vi "Auto Tune.vi"() -> ()   [LabVIEW 2022 SP3]
uses:
  Control_AutoTune.ctl
  <vilib>/Analysis/baseanly.llb/Mean (DBL).vi
  <vilib>/Analysis/NI_AALBase.lvlib
panel:
  in  "Cancel Current Aquisition":bool
  out "XY Graph":cluster{"X":dbl, "Y":dbl}[](graph)=[{"X"=0.0, "Y"=0.49504944043821886}]
  out "Enum":T1
  in  "Channels to read":tag="Dev1/ai2,Dev1/ai3"
  in  "Time per aquisition (s)":dbl
  in  "Sampling Rate":dbl
  out "Best Value":dbl
  out "Max":dbl=0.49504944043821886
  in  "Increment Amount":dbl=5.0
  in  "Lower Value":dbl
  in  "Upper Value":dbl=1000.0
  in  "Start Auto Tune":bool
  in  "stop":bool
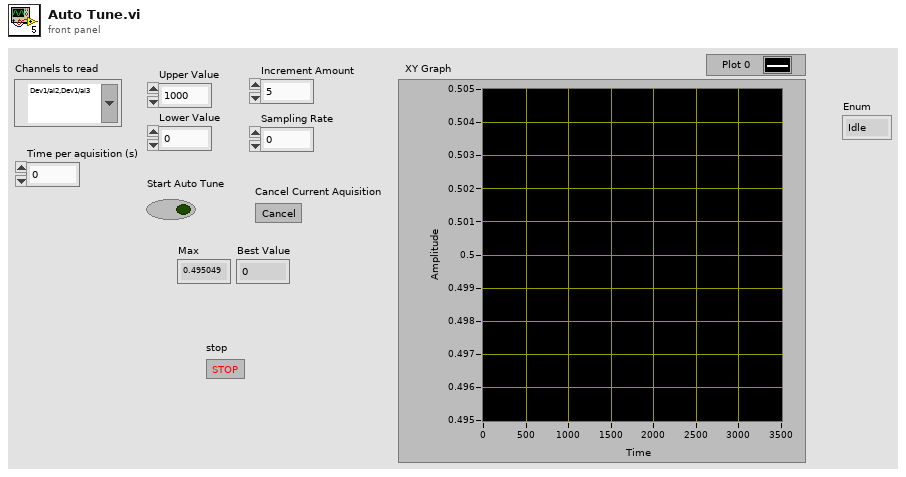
[diagram p1: front panel]
types:
  T1 = typedef "Control_AutoTune.ctl" = enum16{"Idle", "Read DAQ and Store ", "Move to Next Point", "Auto Tune"}
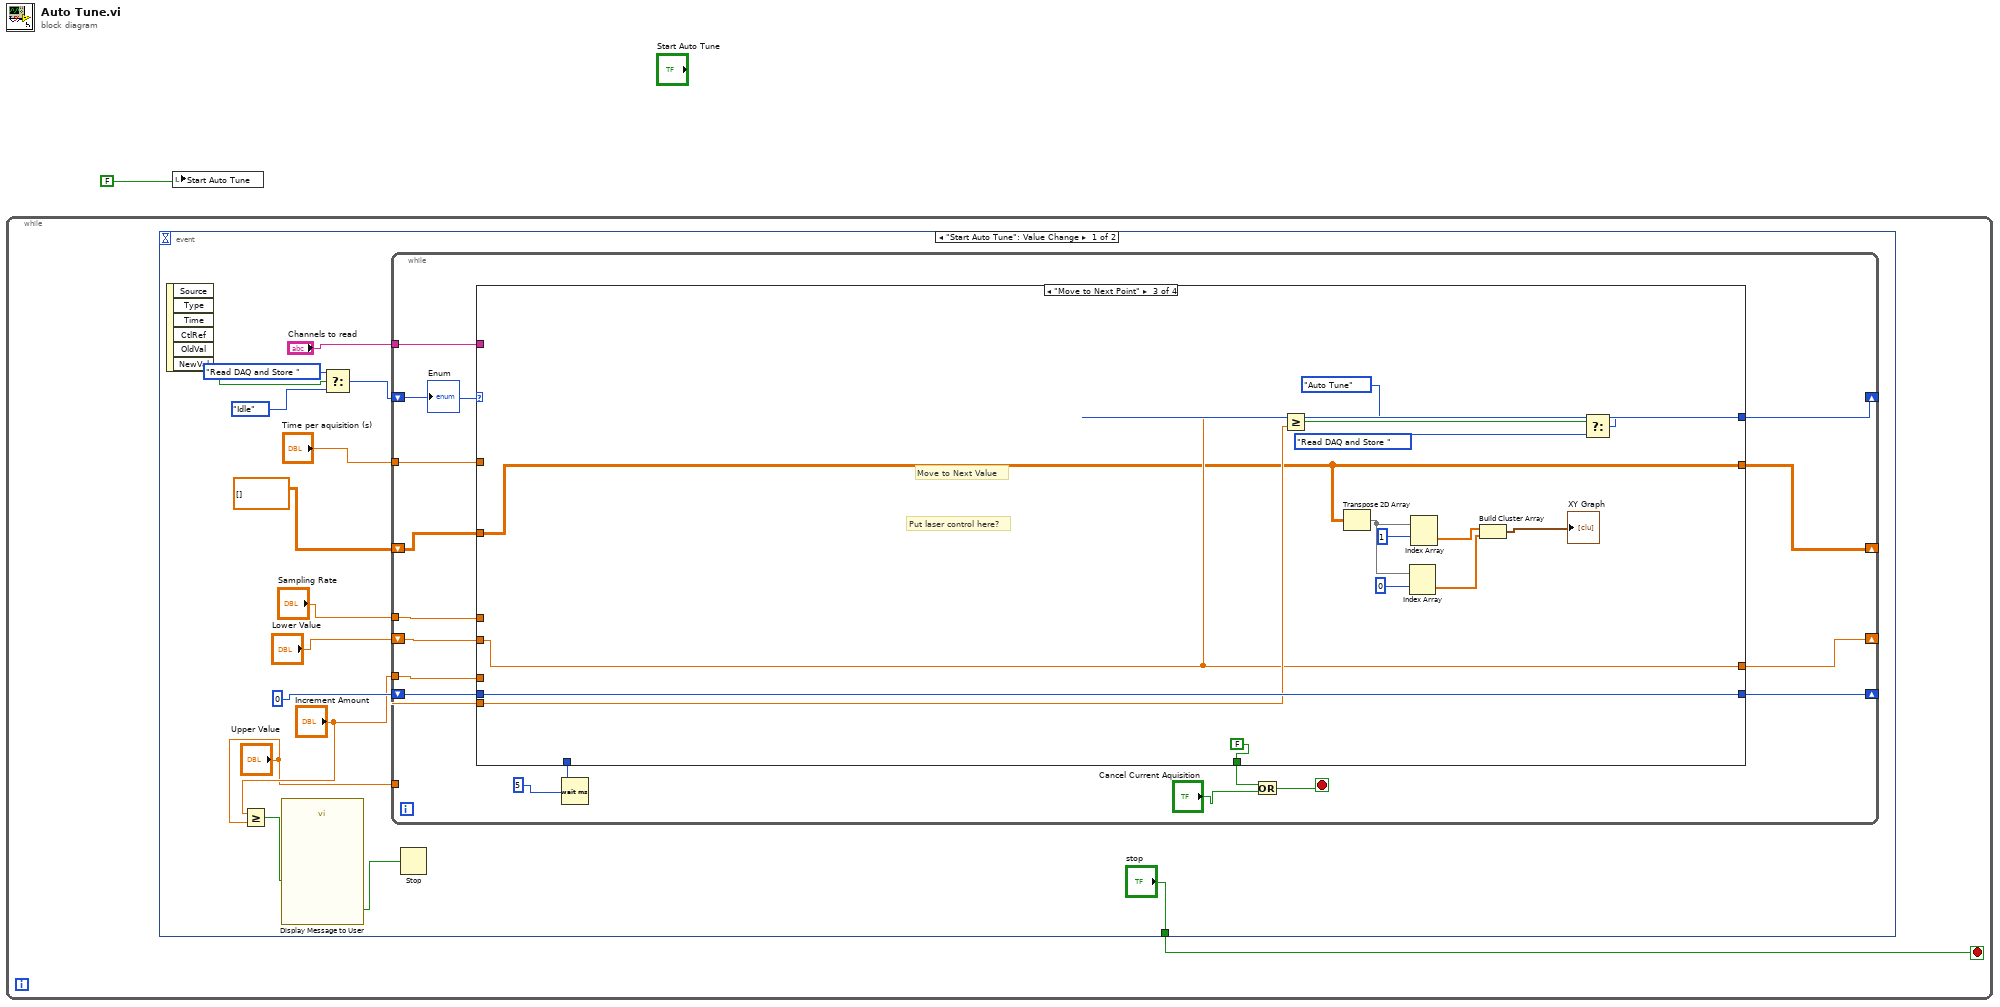
[diagram p0: block diagram]
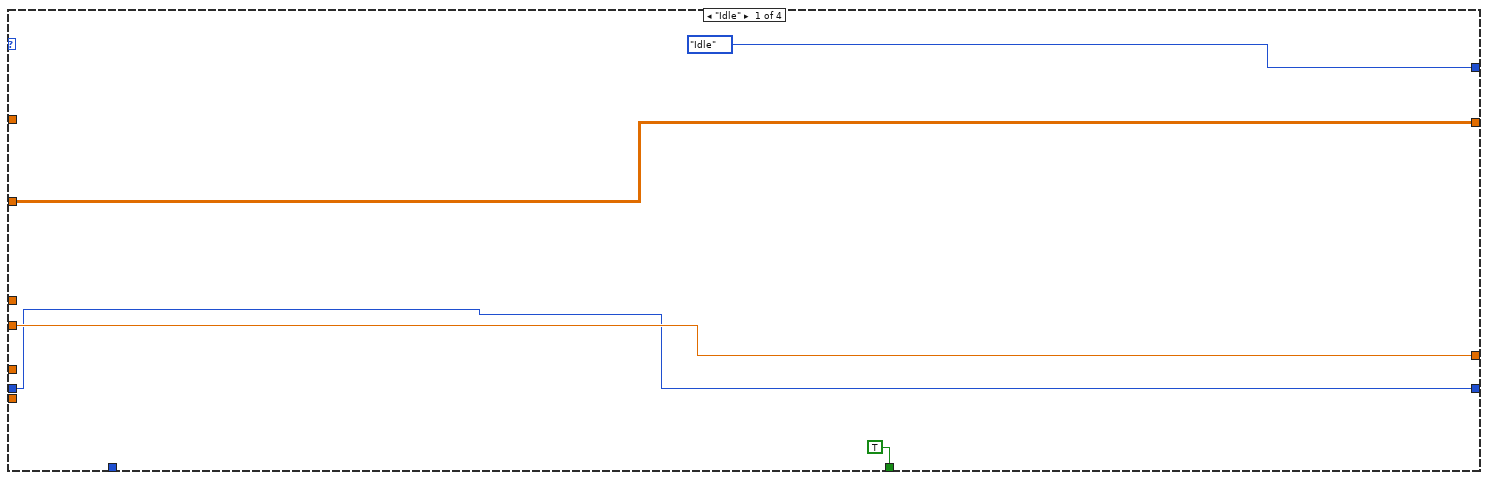
[diagram p2: hidden frame]
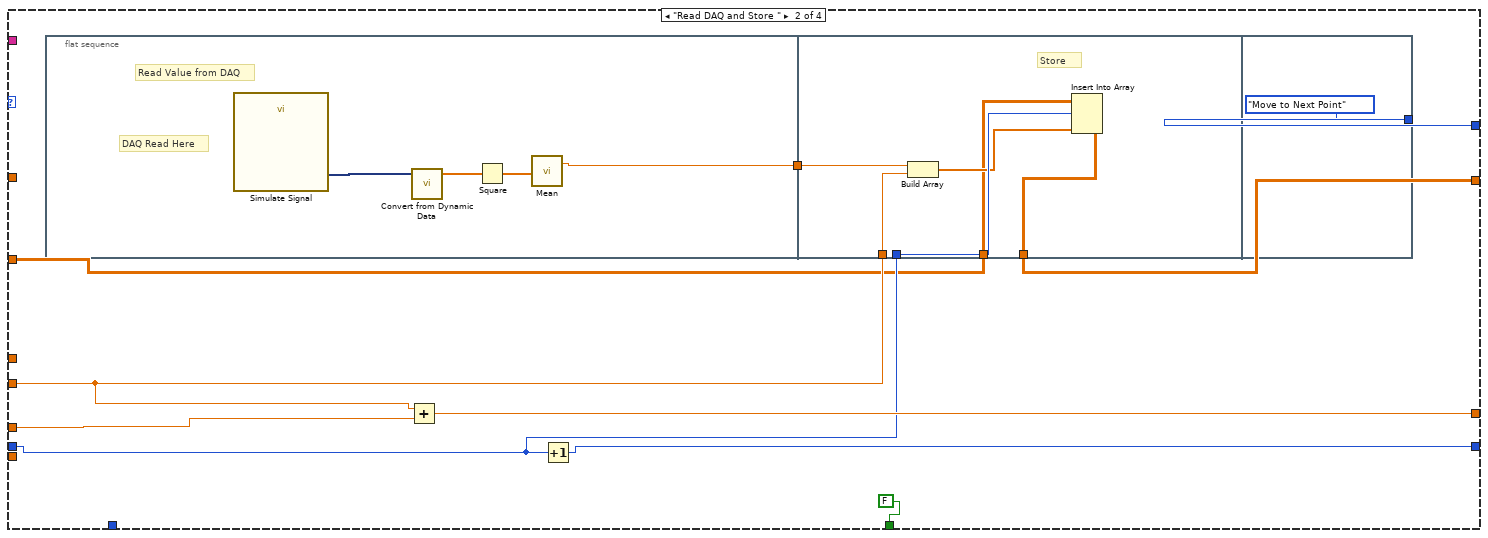
[diagram p3: hidden frame]
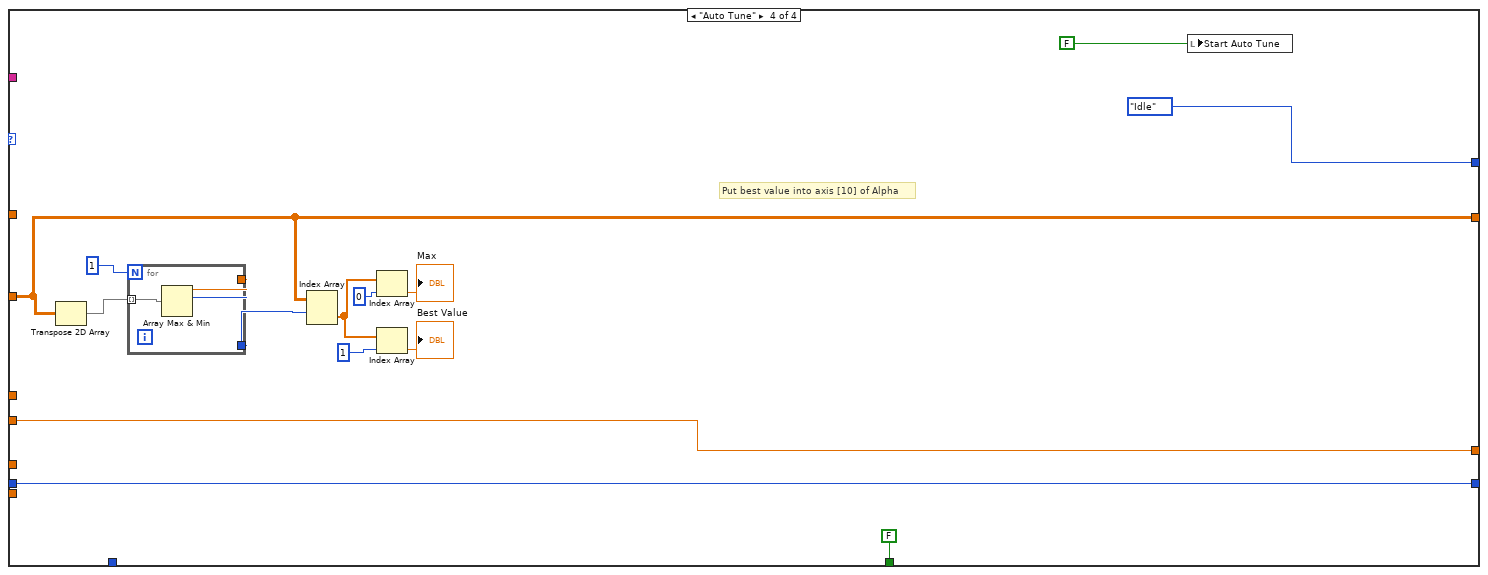
[diagram p4: hidden frame]
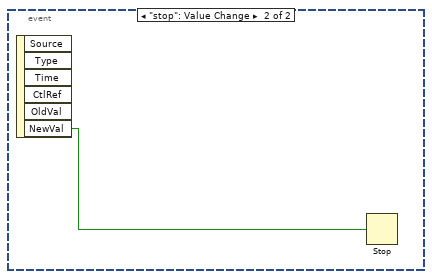
[diagram p5: hidden frame]
diagram:
  n1 = while {
    stop <- w2 stop-if-true
    n2 = event shown="[0] \"Start Auto Tune\": Value Change" {
      selector: _ -> [_ _]
      dyn-events: _ -> [_ _]
      timeout: _ -> [_ _]
      tunnel: ["stop" _] -> w2
      event "Start Auto Tune": Value Change {
        n3 = event-data() -> ("NewVal"=w7:bool)  [unwired: 1 in, 5 out]
        n4 = Greater Or Equal?(x="Increment Amount", y="Upper Value") -> (x >= y?=w6:bool)
        n5 = call "Display Message to User"("Enable"=w6) -> ("OK"=w11:bool)  [unwired: 9 in, 1 out]
        n6 = Select(t=Control_AutoTune."Read DAQ and Store ", s=w7, f=Control_AutoTune."Idle") -> (s? t:f=w8:T1)
        n7 = while {
          shift-right: [w34] -> _
          shift-left: w8 -> [w25]
          shift-right: [w32] -> _
          shift-left: dbl[][] [] -> [w31]
          tunnel: "Increment Amount" -> [w30]
          tunnel: "Upper Value" -> [w21]
          tunnel: "Time per aquisition (s)" -> [w28]
          tunnel: "Sampling Rate" -> [w27]
          tunnel: "Channels to read" -> [w26]
          shift-right: [w24] -> _
          shift-left: 0 -> [w23]
          shift-right: [w22] -> _
          shift-left: "Lower Value" -> [w29]
          stop <- w19 stop-if-true
          w33 = 5
          n8 = case shown="\"Move to Next Point\"" w25 {
            tunnel: [Control_AutoTune."Idle" w46 w72 Control_AutoTune."Idle"] -> w34
            tunnel: w33 -> [_ _ _ _]
            tunnel: [w39 w40 w65 w84] -> w32
            tunnel: w31 -> [w39 w41 w65 w84]
            tunnel: w30 -> [_ w49 _ _]
            tunnel: w29 -> [w38 w47 w69 w77]
            tunnel: w28 -> [_ _ _ _]
            tunnel: w27 -> [_ _ _ _]
            tunnel: w26 -> [_ _ _ _]
            tunnel: [w35 w44 w75 w78] -> w24
            tunnel: w23 -> [w35 w42 w75 w78]
            tunnel: [w38 w45 w69 w77] -> w22
            tunnel: w21 -> [_ _ w70 _]
            tunnel: [TRUE FALSE FALSE FALSE] -> w20
            frame "Idle" {
            }
            frame "Read DAQ and Store " {
              n9 = flat-sequence {
                tunnel: [w53] -> w48
                tunnel: w48 -> [w59]
                tunnel: w47 -> [w58]
                tunnel: w42 -> [w57]
                tunnel: w41 -> [w55]
                tunnel: [w54] -> w40
                tunnel: [Control_AutoTune."Move to Next Point"] -> w46
                frame #0 {
                  # "DAQ Read Here"
                  # "Read Value from DAQ"
                  n10 = call "Simulate Signal"() -> ("Sine"=w52:dynamicdata)  [unwired: 14 in, 1 out]
                  n11 = call "Convert from Dynamic Data"("Dynamic Data Type"=w52) -> ("Array"=w51:dbl[])  [unwired: 3 in]
                  n12 = Square(x=w51) -> (x^2=w50:dbl[])
                  n13 = call-poly <vilib>:"Mean.vi"("X"=w50) -> ("mean"=w53:dbl)  [unwired: 1 out]
                }
                frame #1 {
                  # "Store"
                  n14 = Build Array(w59, w58) -> (w56:dbl[])
                  n15 = Insert Into Array(array=w55, index (row)=w57, new element=w56) -> (w54:dbl[][])  [unwired: 1 in]
                }
                frame #2 {
                }
              }
              n16 = Add(x=w47, y=w49) -> (x+y=w45:dbl)
              n17 = Increment(x=w42) -> (x+1=w44:i32)
            }
            frame "Move to Next Point" {
              # "Put laser control here?"
              # "Move to Next Value"
              n18 = Greater Or Equal?(x=w69, y=w70) -> (x >= y?=w71:bool)
              n19 = Transpose 2D Array(2D array=w65) -> (transposed array=w63:dbl[][])
              n20 = Index Array(array=w63, index (row)=0) -> (element=w62:dbl[])  [unwired: 1 in]
              n21 = Index Array(array=w63, index (row)=1) -> (element=w67:dbl[])  [unwired: 1 in]
              n22 = Build Cluster Array(w67, w62) -> (→"XY Graph":cluster{dbl, dbl}[])
              n23 = Select(t=Control_AutoTune."Auto Tune", s=w71, f=Control_AutoTune."Read DAQ and Store ") -> (s? t:f=w72:T1)
            }
            frame "Auto Tune" {
              # "Put best value into axis [10] of Alpha"
              n24 = Transpose 2D Array(2D array=w84) -> (transposed array=w86:dbl[][])
              n25 = for {
                N: 1 -> [_]
                tunnel: w86 -> [w92] mode=indexing
                tunnel: [w91] -> w85
                tunnel: [w90] -> _
                n26 = Array Max & Min(array=w92) -> (max value=w90:dbl, max index (indices)=w91:i32)  [unwired: 2 out]
              }
              n27 = Index Array(array=w84, index (row)=w85) -> (element=w83:dbl[])  [unwired: 1 in]
              n28 = Index Array(array=w83, index=0) -> (element=→"Max":dbl)
              n29 = Index Array(array=w83, index=1) -> (element=→"Best Value":dbl)
              n30 = local write "Start Auto Tune"(FALSE) -> ()
            }
          }
          n31 = Wait (ms)(milliseconds to wait=w33) -> ()  [unwired: 1 out]
          n32 = Or(x=w20, y="Cancel Current Aquisition") -> (x .or. y?=w19:bool)
          "Enum" <- w25
        }
        n33 = Stop(stop? (T)=w11) -> ()
      }
      event "stop": Value Change {
        n34 = event-data() -> ("NewVal"=w93:bool)  [unwired: 1 in, 5 out]
        n35 = Stop(stop? (T)=w93) -> ()
      }
    }
  }
  n36 = local write "Start Auto Tune"(FALSE) -> ()
